vi "uActor_Cleanup.vi"(8 "error in (no error)":errorcluster, 11 "uActor in":refnum<class "uActor.lvclass">) -> (0 "error out":errorcluster, 3 "uActor out":refnum<class "uActor.lvclass">)   [LabVIEW 2023, in "uLib.lvlib" / "uActor.lvclass"]
doc: "Dynamic dispatch method that is called when the actor is stopping. This allows children to extend the shutdown routine.\nThe default behavior of the parent is to send a stop msg to all nested actors and wait for confirmation that they all stopped.\n\n<B>Children must call the parent method.</B>"
uses:
  uActor.lvclass
  uActor.lvclass/uActor.ctl
  uMsg/uMsg/uMsg.lvclass/uMsg.ctl
  uTransport/uTransport_uActor/uTransport_uActor.lvclass/uTransport_uActor.ctl
  uActor_CMDs_Prefix.vi
  uActor_SimpleSend.vi
  uActor_SendMsg.vi
  uMsg/uMsg/uMsg Create.vi
  uTransport/uTransport_uActor/uTransport_uActor_SendMsg.vi
  uMsg/uMsg/uMsg Update Timestamp.vi
  uData/uData/uData.lvclass
  uTransport/uTransport/uTransport.lvclass
  uMsg/uMsg/uMsg.lvclass
  uTransport/uTransport_uActor/uTransport_uActor.lvclass
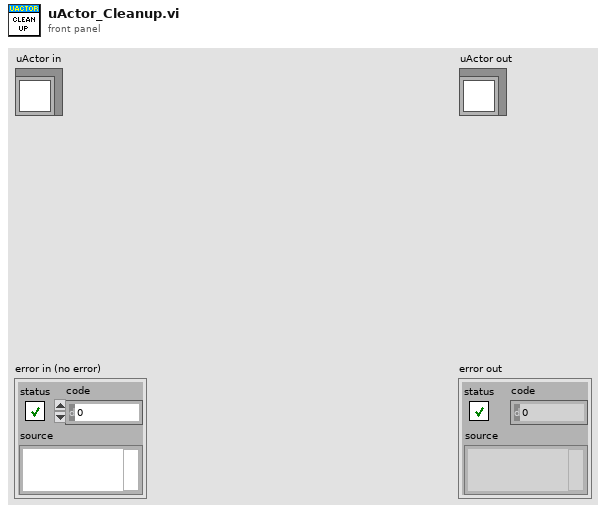
[diagram p1: front panel]
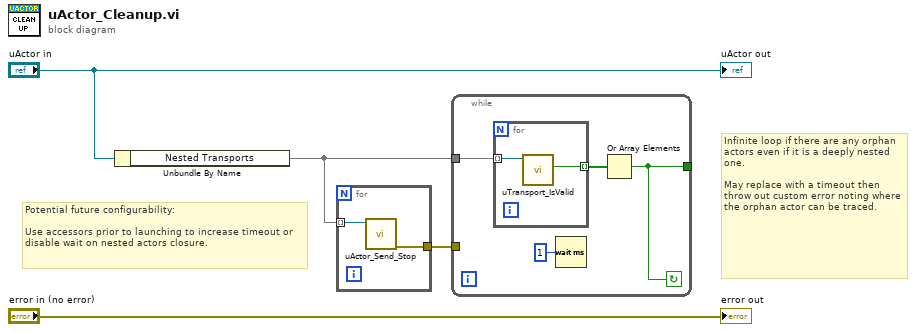
[diagram p0: block diagram]
diagram:
  # "Infinite loop if there are any orphan actors even if it is a deeply nested one.\n\nMay replace with a timeout then throw out custom error noting where the orphan actor can be traced."
  # "Potential future configurability:\n\nUse accessors prior to launching to increase timeout or disable wait on nested actors closure."
  n1 = Unbundle By Name("uActor in") -> ("Nested Transports"=w1:set{refnum<class "uTransport_uActor.lvclass">})
  n2 = for {
    tunnel: w1 -> [w6] mode=indexing
    tunnel: [w5] -> w2
    n3 = call "uActor_Send_Stop.vi"("uActor Transport"=w6) -> ("error out"=w5:errorcluster)  [unwired: 10 in]
  }
  n4 = while {
    tunnel: w2 -> [_]
    tunnel: w1 -> [w10]
    tunnel: [w8] -> _
    stop <- w8 continue-if-true
    n5 = for {
      tunnel: w10 -> [w12] mode=indexing
      tunnel: [w11] -> w9 mode=indexing
      n6 = call-dynamic "uTransport_IsValid.vi"("uTransport_uActor in"=w12) -> ("IsValid?"=w11:bool)  [unwired: 8 in, 2 out]
    }
    n7 = Wait (ms)(milliseconds to wait=u32 1) -> ()  [unwired: 1 out]
    n8 = Or Array Elements(Boolean array=w9) -> (logical OR=w8:bool)
  }
  "error out" <- "error in (no error)"
  "uActor out" <- "uActor in"
